vi "Generate Error Codes Text File from Spreadsheet.vi"() -> ()   [LabVIEW 2015]
uses:
  <vilib>/addons/_office/excel.llb/Excel Get Data ([str]).vi
  <vilib>/Utility/NIReport.llb/NI_report.lvclass
  <vilib>/addons/_office/NI_ReportGenerationToolkit.lvlib
  <vilib>/Utility/NIReport.llb/Excel/NI_Excel.lvclass
panel:
  out "error out":errorcluster
  out "TXT file contents":string
  out "Resulting Error Codes TXT file":path
  in  "Error Codes Spreadsheet":path
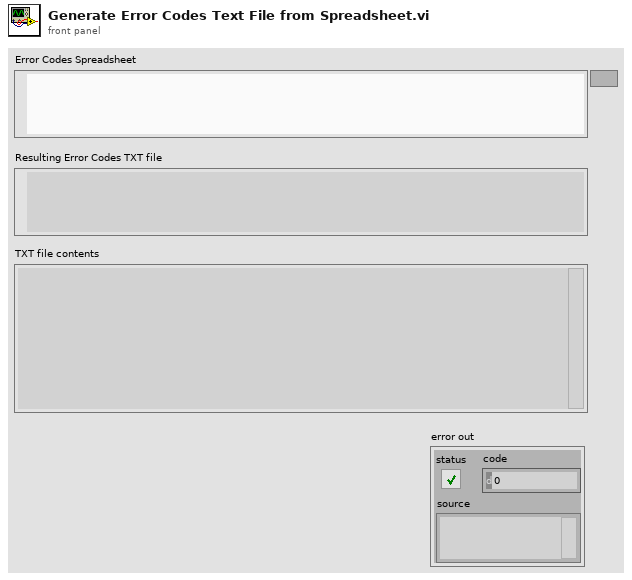
[diagram p1: front panel]
types:
  T1 = enum16{"Standard Report", "HTML", "Word", "Excel"}
  T2 = enum16{"maximized", "minimized", "normal", "no change"}
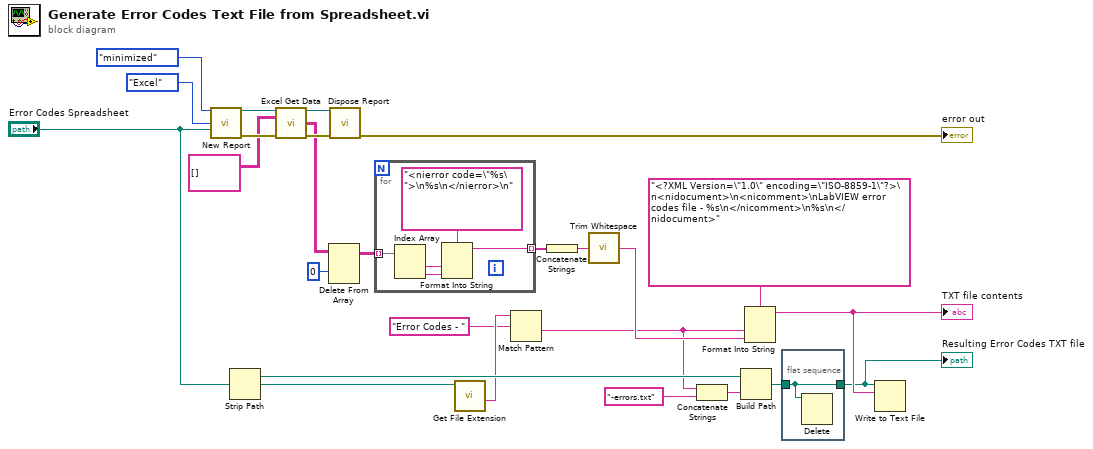
[diagram p0: block diagram]
diagram:
  n1 = call <vilib>:"New Report.vi"("window state (normal)"=T2."minimized", "report type"=T1."Excel", "template (empty)"="Error Codes Spreadsheet") -> ("report out"=w23:refnum<class "NI_report.lvclass">, "error out"=w22:errorcluster)  [unwired: 11 in]
  n2 = Strip Path(path="Error Codes Spreadsheet") -> (stripped path=w13:path)  [unwired: 1 out]
  n3 = call-poly <vilib>:"Excel Get Data.vi"("report in"=w23, "data type"=string[][] [], "error in (no error)"=w22) -> ("report out"=w20:refnum<class "NI_report.lvclass">, "data"=w9:string[][], "error out"=w19:errorcluster)  [unwired: 10 in]
  n4 = Delete From Array(array=w9, index (row)=0) -> (array with subset deleted=w7:string[][])  [unwired: 2 in, 1 out]
  n5 = call-dynamic "Dispose Report.vi"("report in"=w20, "error in (no error)"=w19) -> ("error out"=→"error out":errorcluster)  [unwired: 13 in]
  n6 = for {
    tunnel: w7 -> [w29] mode=indexing
    tunnel: [w26] -> w6 mode=indexing
    n7 = Index Array(array=w29) -> (element #1=w28:string, element #2=w27:string)  [unwired: 2 in]
    n8 = Format Into String(format string="<nierror code=\"%s\">\n%s\n</nierror>\n", w28, w27) -> (resulting string=w26:string)  [unwired: 2 in, 1 out]
  }
  n9 = call <vilib>:"Get File Extension.vi"("file"="Error Codes Spreadsheet") -> ("filename without extension"=w3:string)  [unwired: 6 in, 4 out]
  n10 = Match Pattern(string=w3, regular expression="Error Codes - ") -> (after substring=w2:string)  [unwired: 1 in, 3 out]
  n11 = Concatenate Strings(w6) -> (w5:string)
  n12 = call <vilib>:"Trim Whitespace.vi"("string"=w5) -> ("trimmed string"=w4:string)  [unwired: 1 in]
  n13 = Concatenate Strings(w2, "-errors.txt" ("string")) -> (w14:string)
  n14 = Build Path(base path=w13, name or relative path=w14) -> (appended path=w11:path)
  n15 = Format Into String(format string="<?XML Version=\"1.0\" encoding=\"ISO-8859-1\"?>\n<nidocument>\n<nicomment>\nLabVIEW error codes file - %s\n</nicomment>\n%s\n</nidocument>", w2, w4) -> (resulting string=w12:string)  [unwired: 2 in, 1 out]
  "TXT file contents" <- w12
  n16 = flat-sequence {
    tunnel: w11 -> [w31]
    tunnel: [w31] -> w10
    frame #0 {
      n17 = Delete(path (use dialog)=w31) -> ()  [unwired: 4 in, 3 out]
    }
  }
  n18 = Write to Text File(file (use dialog)=w10, text=w12) -> ()  [unwired: 2 in, 3 out]
  "Resulting Error Codes TXT file" <- w10
